vi "Configure Auto Frequency.vi"(0 "VISA resource name":refnum<visa-resource-name>, 1 "Maximum Iterations (10)":i32=10, 2 "Tuning Sensitivity (10E6 Hz/V)":dbl=10000000.0 format="%^#_9g", 3 "Min Control Voltage Limit (-15 V)":dbl=-15.0 format="%^#_9g", 5 "Maximum Input Level (0 dBm)":dbl format="%^#_9g", 7 "Auto Frequency Control Mode (2: Off)":u16(ring)=2 items=["On", "Immediate", "Off"], 9 "Tolerance Frequency (1E3 Hz)":dbl=1000.0 format="%^#_9g", 11 "error in (no error)":errorcluster, 12 "Target Frequency (1E9 Hz)":dbl=1000000000.0 format="%^#_9g", 13 "Max Control Voltage Limit (35 V)":dbl=35.0 format="%^#_9g") -> (4 "VISA resource name out":refnum<visa-resource-name>, 15 "error out":errorcluster)   [LabVIEW 2011, in "Agilent E5052X.lvlib"]
doc: "Configures the Automatic Frequency Control function. The Automatic Frequency Control (AFC) function can quickly set and maintain the Device Under Test (DUT) output frequency to the target frequency you want. It does this by controlling the internal DC control voltage and using the measurement results obtained by its internal frequency counter. \n\n<b>Note: </b>\n\nThe DC control voltage has to be turned on to use the AFC function.\n\n<b>Note: </b>\n\n1) The AFC starts immediately before the measurement. During a single measurement, the DC control voltage is maintained. Therefore, the DC control voltage will not be changed even if the actual output frequency from the DUT drifts during the measurement.\n\n2) When the external mixer is set to OFF, the auto frequency control function is not available."
uses:
  Agilent E5052X.lvlib
panel:
  # "Auto Frequency Control Settings"
  # "Control Voltage Settings"
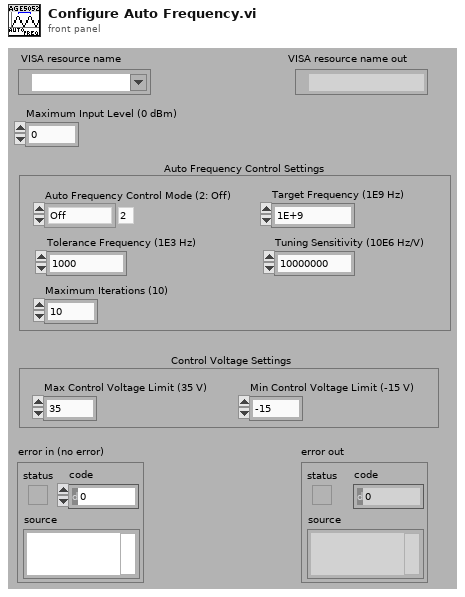
[diagram p1: front panel]
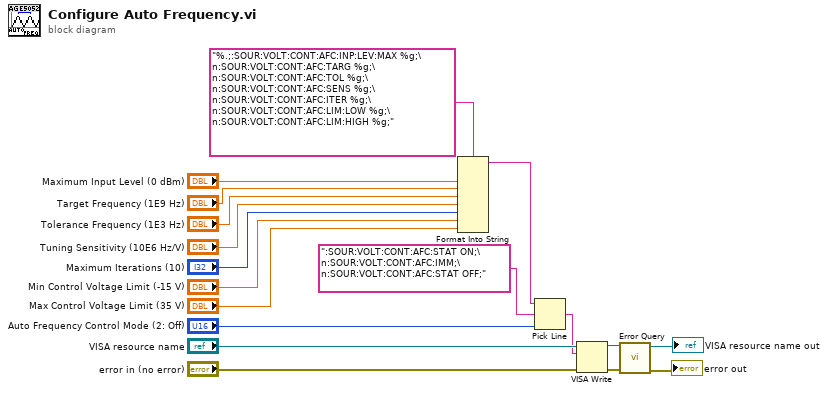
[diagram p0: block diagram]
diagram:
  n1 = Format Into String(format string="%.;:SOUR:VOLT:CONT:AFC:INP:LEV:MAX %g;\n:SOUR:VOLT:CONT:AFC:TARG %g;\n:SOUR:VOLT:CONT:AFC:TOL %g;\n:SOUR:VOLT:CONT:AFC:SENS %g;\n:SOUR:VOLT:CONT:AFC:ITER %g;\n:SOUR:VOLT:CONT:AFC:LIM:LOW %g;\n:SOUR:VOLT:CONT:AFC:LIM:HIGH %g;", "Maximum Input Level (0 dBm)", "Target Frequency (1E9 Hz)", "Tolerance Frequency (1E3 Hz)", "Tuning Sensitivity (10E6 Hz/V)", "Maximum Iterations (10)", "Min Control Voltage Limit (-15 V)", "Max Control Voltage Limit (35 V)") -> (resulting string=w2:string)  [unwired: 2 in, 1 out]
  n2 = Pick Line(string ("")=w2, multi-line string=":SOUR:VOLT:CONT:AFC:STAT ON;\n:SOUR:VOLT:CONT:AFC:IMM;\n:SOUR:VOLT:CONT:AFC:STAT OFF;", line index="Auto Frequency Control Mode (2: Off)") -> (output string=w1:string)
  n3 = VISA Write(VISA resource name="VISA resource name", write buffer=w1, error in (no error)="error in (no error)") -> (VISA resource name out=w8:refnum<visa-resource-name>, error out=w7:errorcluster)  [unwired: 1 out]
  n4 = call "Error Query.vi"("error in (no error)"=w7, "VISA resource name"=w8) -> ("error out"=→"error out":errorcluster, "VISA resource name out"=→"VISA resource name out":refnum<visa-resource-name>)  [unwired: 6 in, 2 out]
